vi "Begin.vi"(8 "error in":errorcluster) -> (0 "error out":errorcluster)   [LabVIEW 2014]
doc: "Called before other user functions, this VI is expected to open initial I/O refnums, load in file data, and do all program initialization. Notice that the <B>error out</B> terminal is simply used for data flow. Wiring it to other structures or subVIs ensures that this VI runs first."
uses:
  <vilib>/Rock Robotics/WPI/DriverStation/WPI_DriverStationRobotMode2.ctl
  <vilib>/Rock Robotics/SystemInterfaces/DIO/FPGA_DIOPWMChannel.ctl
  <vilib>/Rock Robotics/WPI/SafetyOutput/WPI_SafetyOutputConfigMenu.ctl
  <vilib>/Rock Robotics/WPI/Joystick/WPI_JoystickDeviceEnum.ctl
  <vilib>/Rock Robotics/SystemInterfaces/DIO/FPGA_DIOChannel.ctl
  <vilib>/Rock Robotics/SystemInterfaces/Typedef/FPGA_TypedefAnalogModuleForGyro.ctl
  <vilib>/Rock Robotics/SystemInterfaces/AI/FPGA_AIGyroChannel.ctl
  <vilib>/Rock Robotics/WPI/Solenoid/WPI_SolenoidChannel.ctl
  <vilib>/Rock Robotics/Network Tables/SD Write String Array.vi
  Robot Global Data.vi
  <vilib>/Rock Robotics/WPI/MotorControl/WPI_MotorControlOpen Talon.vi
  <vilib>/Rock Robotics/WPI/RobotDrive/WPI_RobotDriveOpen4MotorWithTalon.vi
  <vilib>/Rock Robotics/WPI/Counter/WPI_CounterDigitalInputToDigitalSource.vi
  <vilib>/Rock Robotics/WPI/Solenoid/WPI_SolenoidOpenSingle.vi
  <vilib>/Rock Robotics/WPI/Solenoid/WPI_SolenoidOpenDouble.vi
  <vilib>/Rock Robotics/WPI/Compressor/WPI_CompressorGetSetRefNum.vi
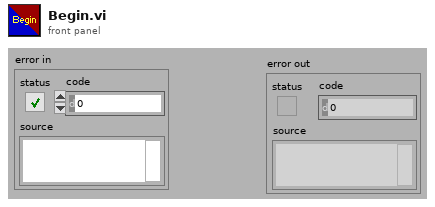
[diagram p1: front panel]
types:
  T1 = typedef "WPI_SolenoidChannel.ctl" = enum8{"Solenoid 0", "Solenoid 1", "Solenoid 2", "Solenoid 3", "Solenoid 4", "Solenoid 5", "Solenoid 6", "Solenoid 7", "Invalid"}
  T2 = typedef "FPGA_DIOChannel.ctl" = enum8{"DIO 0", "DIO 1", "DIO 2", "DIO 3", "DIO 4", "DIO 5", "DIO 6", "DIO 7", "DIO 8", "DIO 9", "DIO MXP 0", "DIO MXP 1", "DIO MXP 2", "DIO MXP 3", "DIO MXP 4", "DIO MXP 5", "DIO MXP 6", "DIO MXP 7", "DIO MXP 8", "DIO MXP 9", "DIO MXP 10", "DIO MXP 11", "DIO MXP 12", "DIO MXP 13", "DIO MXP 14", "DIO MXP 15", "Invalid"}
  T3 = typedef "FPGA_DIOPWMChannel.ctl" = enum8{"PWM 0", "PWM 1", "PWM 2", "PWM 3", "PWM 4", "PWM 5", "PWM 6", "PWM 7", "PWM 8", "PWM 9", "PWM MXP 0", "PWM MXP 1", "PWM MXP 2", "PWM MXP 3", "PWM MXP 4", "PWM MXP 5", "PWM MXP 6", "PWM MXP 7", "PWM MXP 8", "PWM MXP 9", "Invalid"}
  T4 = typedef "FPGA_AIGyroChannel.ctl" = enum8{"AI 0", "AI 1", "Invalid"}
  T5 = typedef "FPGA_TypedefAnalogModuleForGyro.ctl" = enum16{"Controller 1"}
  T6 = typedef "WPI_JoystickDeviceEnum.ctl" = enum16{"USB 0", "USB 1", "USB 2", "USB 3", "USB 4", "USB 5"}
  T7 = typedef "WPI_SafetyOutputConfigMenu.ctl" = enum16{"Enable", "Disable"}
  T8 = typedef "WPI_DriverStationRobotMode2.ctl" = enum16{"Autonomous Disabled", "Autonomous Enabled", "Teleop Disabled", "Teleop Enabled", "Disconnected", "Finish", "Test Disabled", "Test Enabled", "Emergency Stopped"}
  T9 = typedef "WPI_MotorControlDeviceRef.ctl" = cluster{"DeviceStatus":errorcluster, "Type":T10, "PWM":cluster{"Controller":T11, "PWM Channel":T3, "DeadBand":T12}, "CAN":cluster{"Device Number":u8, "Control Mode":T13, "Semaphore":T14, "Max Vout":dbl, "TalonSRX Control Mode":T15}, "Invert":bool, "TransformRef":T16, "InvTransformRef":T16}
  T10 = typedef "WPI_MotorControlType.ctl" = enum16{"PWM", "CAN", "CANTalonSRX"}
  T11 = typedef "FPGA_TypedefDigitalModule.ctl" = enum16{"Controller 1"}
  T12 = typedef "WPI_PWMDeadband.ctl" = cluster{"Name":string, "maxPositivePwm":i32, "minPositivePwm":i32, "centerPwm":i32, "maxNegativePwm":i32, "minNegativePwm":i32, "angularRange":u16}
  T13 = typedef "WPI_CANJaguar_ControlMode.ctl" = enum8{"Percent VBus", "Current", "Speed", "Position", "Voltage"}
  T14 = typedef "Semaphore RefNum" = refnum<k1>
  T15 = typedef "WPI_CANTalonSRX_APIControlMode.ctl" = enum8{"Percent VBus", "Speed", "Position", "Slave", "Unchanged / Invalid"}
  T16 = typedef "WPI_PWMTransform_ConPane.ctl" = refnum<vi>
  T17 = typedef "WPI_CompressorDevRef.ctl" = cluster{"DevStatus":errorcluster, "Pneumatics Control Module":u8}
  T18 = typedef "WPI_DigitalInputDevRef.ctl" = cluster{"DevStatus":errorcluster, "DIO Channel":T2, "Controller":T11}
  T19 = typedef "WPI_JoystickDevRef.ctl" = cluster{"Device":T6}
  T20 = typedef "WPI_SolenoidDevRef.ctl" = cluster{"DevStatus":errorcluster, "Pneumatics Control Module":u8, "Forward Solenoid Channel":T1, "Reverse Solenoid Channel":T1}
  T21 = typedef "WPI_GyroDevRef.ctl" = cluster{"DevStatus":errorcluster, "Analog Module":T22, "Analog Channel":T23, "Offset":dbl, "Gain (VoltsPerDegree/Second)":dbl}
  T22 = typedef "FPGA_TypedefAnalogModule.ctl" = enum16{"Controller 1"}
  T23 = typedef "FPGA_AIChannel.ctl" = enum8{"AI 0", "AI 1", "AI 2", "AI 3", "AI MXP 0", "AI MXP 1", "AI MXP 2", "AI MXP 3", "Invalid"}
  T24 = typedef "FPGA_CounterEncoderSourceConvertionLVSourceType.ctl" = cluster{"DevStatus":errorcluster, "AnalogTriggerMode?":bool, "DigitalMode":cluster{"Controller":T11, "DIO Channel":T25}, "AnalogTriggerMode":cluster{"AnalogTriggerIndex":T26, "OutputType":T27}}
  T25 = typedef "FPGA_DIODigitalSourceChannel.ctl" = enum8{"DIO 0", "DIO 1", "DIO 2", "DIO 3", "DIO 4", "DIO 5", "DIO 6", "DIO 7", "DIO 8", "DIO 9", "DIO MXP 0", "DIO MXP 1", "DIO MXP 2", "DIO MXP 3", "DIO MXP 4", "DIO MXP 5", "DIO MXP 6", "DIO MXP 7", "DIO MXP 8", "DIO MXP 9", "DIO MXP 10", "DIO MXP 11", "DIO MXP 12", "DIO MXP 13", "DIO MXP 14", "DIO MXP 15", "Disabled"}
  T26 = typedef "FPGA_AnalogTriggerIndex.ctl" = enum8{"Trig 0", "Trig 1", "Trig 2", "Trig 3", "Trig 4", "Trig 5", "Trig 6", "Trig 7", "Invalid"}
  T27 = typedef "FPGA_AnalogTriggerOutType.ctl" = enum16{"InWindow", "TriggerState", "Rising", "Falling"}
  T28 = typedef "WPI_RobotDriveDevRef.ctl" = cluster{"DevStatus":errorcluster, "Motors[]":T9[], "Square Inputs":bool, "Max Output":dbl}
  T29 = typedef "WPI_EncoderDevRef.ctl" = cluster{"DevStatus":errorcluster, "EncoderIndex":T30, "CounterIndex":T31, "DistancePerCount":dbl, "Decoding Type":T32}
  T30 = typedef "FPGA_EncoderIdx.ctl" = enum8{"Enc 0", "Enc 1", "Enc 2", "Enc 3", "Enc 4", "Enc 5", "Enc 6", "Enc 7", "Invalid"}
  T31 = typedef "FPGA_CounterCtrSystemIndex.ctl" = enum8{"Ctr 0", "Ctr 1", "Ctr 2", "Ctr 3", "Ctr 4", "Ctr 5", "Ctr 6", "Ctr 7", "Invalid"}
  T32 = typedef "WPI_EncoderType.ctl" = enum16{"1x", "2x", "4x"}
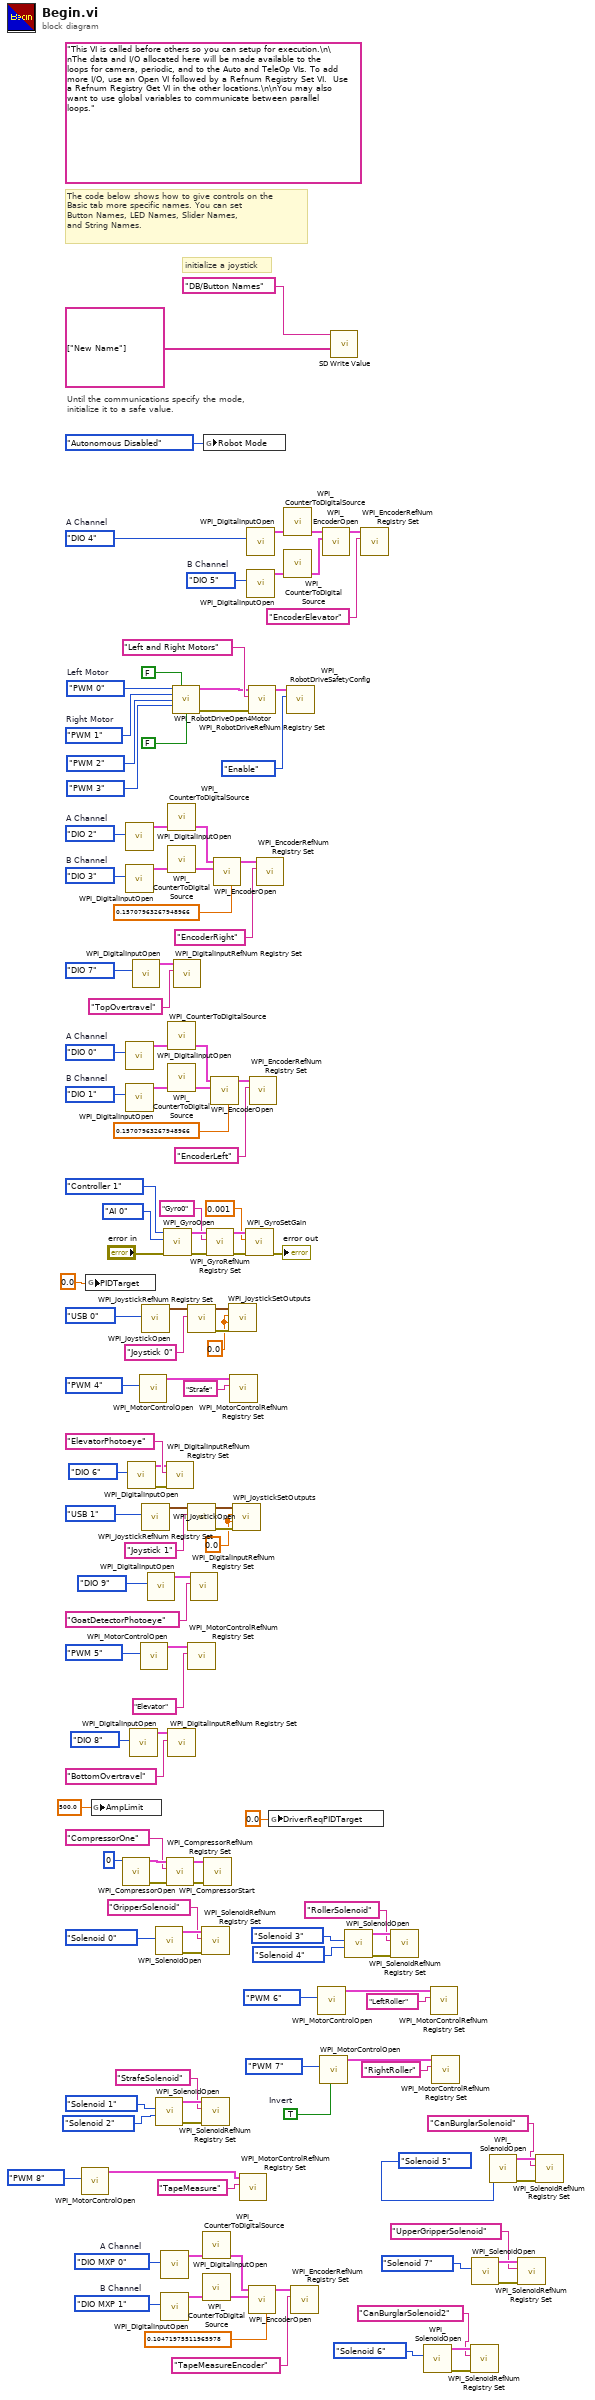
[diagram p0: block diagram]
diagram:
  w10 = 0.0
  w11 = 0.0
  w20 = FPGA_DIOChannel."DIO MXP 1"  # B Channel
  w21 = FPGA_DIOChannel."DIO MXP 0"  # A Channel
  w31 = TRUE  # Invert
  w118 = FPGA_DIOChannel."DIO 5"  # B Channel
  w119 = FPGA_DIOChannel."DIO 4"  # A Channel
  w111 = FPGA_DIOChannel."DIO 3"  # B Channel
  w112 = FPGA_DIOChannel."DIO 2"  # A Channel
  w103 = FPGA_DIOChannel."DIO 1"  # B Channel
  w104 = FPGA_DIOChannel."DIO 0"  # A Channel
  w84 = FPGA_DIOPWMChannel."PWM 1"  # Right Motor
  w83 = FPGA_DIOPWMChannel."PWM 0"  # Left Motor
  (unwired) "This VI is called before others so you can setup for execution.\n\nThe data and I/O allocated here will be made available to the loops for camera, periodic, and to the Auto and TeleOp VIs. To add more I/O, use an Open VI followed by a Refnum Registry Set VI.  Use a Refnum Registry Get VI in the other locations.\n\nYou may also want to use global variables to communicate between parallel loops."
  # "The code below shows how to give controls on the\nBasic tab more specific names. You can set\nButton Names, LED Names, Slider Names,\nand String Names."
  # "initialize a joystick"
  # "Until the communications specify the mode,\ninitialize it to a safe value."
  n1 = call-poly <vilib>:"WPI_MotorControlOpen.vi"("PWM Channel"=FPGA_DIOPWMChannel."PWM 8") -> ("MotorControlDeviceRef"=w28:T9)  [unwired: 9 in, 1 out]
  n2 = global write "Robot Global Data.vi" "PIDTarget"(0.0 ("PIDTarget")) -> ()
  n3 = global write "Robot Global Data.vi" "AmpLimit"(500.0 ("AmpLimit")) -> ()
  n4 = call <vilib>:"WPI_CompressorOpen.vi"("Pneumatics Control Module (0)"=u8 0) -> ("CompressorDevRef"=w62:T17, "error out"=w59:errorcluster)  [unwired: 13 in]
  n5 = call <vilib>:"WPI_DigitalInputOpen.vi"("DIO Channel"=w112) -> ("DigitalInputDevRef"=w115:T18)  [unwired: 2 in, 8 out]
  n6 = call <vilib>:"WPI_DigitalInputOpen.vi"("DIO Channel"=w111) -> ("DigitalInputDevRef"=w114:T18)  [unwired: 2 in, 8 out]
  n7 = call <vilib>:"WPI_DigitalInputOpen.vi"("DIO Channel"=w104) -> ("DigitalInputDevRef"=w107:T18)  [unwired: 2 in, 8 out]
  n8 = call <vilib>:"WPI_DigitalInputOpen.vi"("DIO Channel"=w103) -> ("DigitalInputDevRef"=w106:T18)  [unwired: 2 in, 8 out]
  n9 = call <vilib>:"WPI_DigitalInputOpen.vi"("DIO Channel"=FPGA_DIOChannel."DIO 6") -> ("error out"=w128:errorcluster, "DigitalInputDevRef"=w129:T18)  [unwired: 9 in]
  n10 = call <vilib>:"WPI_DigitalInputOpen.vi"("DIO Channel"=FPGA_DIOChannel."DIO 8") -> ("DigitalInputDevRef"=w67:T18)  [unwired: 9 in, 1 out]
  n11 = call <vilib>:"WPI_DigitalInputOpen.vi"("DIO Channel"=FPGA_DIOChannel."DIO 7") -> ("DigitalInputDevRef"=w69:T18)  [unwired: 9 in, 1 out]
  n12 = call-poly <vilib>:"WPI_MotorControlOpen.vi"("PWM Channel"=FPGA_DIOPWMChannel."PWM 4") -> ("MotorControlDeviceRef"=w93:T9)  [unwired: 9 in, 1 out]
  n13 = call-poly <vilib>:"WPI_MotorControlOpen.vi"("PWM Channel"=FPGA_DIOPWMChannel."PWM 5") -> ("MotorControlDeviceRef"=w98:T9)  [unwired: 9 in, 1 out]
  n14 = call <vilib>:"WPI_JoystickOpen.vi"("JoystickDevice"=WPI_JoystickDeviceEnum."USB 0") -> ("JoystickDevRef"=w88:T19)  [unwired: 10 in]
  n15 = call <vilib>:"WPI_JoystickOpen.vi"("JoystickDevice"=WPI_JoystickDeviceEnum."USB 1") -> ("JoystickDevRef"=w101:T19)  [unwired: 10 in]
  n16 = call <vilib>:"WPI_DigitalInputOpen.vi"("DIO Channel"=FPGA_DIOChannel."DIO 9") -> ("DigitalInputDevRef"=w51:T18)  [unwired: 9 in, 1 out]
  n17 = call-poly <vilib>:"WPI_SolenoidOpen.vi"("Solenoid Channel"=WPI_SolenoidChannel."Solenoid 0") -> ("error out"=w61:errorcluster, "SolenoidDevRef"=w60:T20)  [unwired: 9 in]
  n18 = call-poly <vilib>:"WPI_SolenoidOpen.vi"("Reverse Solenoid Channel"=WPI_SolenoidChannel."Solenoid 2" ("Solenoid Channel"), "Forward Solenoid Channel"=WPI_SolenoidChannel."Solenoid 1" ("Solenoid Channel")) -> ("error out"=w48:errorcluster, "SolenoidDevRef"=w47:T20)  [unwired: 8 in]
  n19 = call <vilib>:"WPI_DigitalInputOpen.vi"("DIO Channel"=w21) -> ("DigitalInputDevRef"=w24:T18)  [unwired: 2 in, 8 out]
  n20 = call <vilib>:"WPI_DigitalInputOpen.vi"("DIO Channel"=w20) -> ("DigitalInputDevRef"=w23:T18)  [unwired: 2 in, 8 out]
  n21 = call <vilib>:"WPI_GyroOpen.vi"("error in (no error)"="error in", "Analog Channel"=FPGA_AIGyroChannel."AI 0", "Controller"=FPGA_TypedefAnalogModuleForGyro."Controller 1") -> ("error out"=w77:errorcluster, "GyroDevRef"=w76:T21)  [unwired: 6 in, 1 out]
  n22 = call <vilib>:"WPI_DigitalInputRefNum Registry Set.vi"("error in (no error)"=w128, "refnum name"="ElevatorPhotoeye", "DigitalInputDevRef"=w129) -> ()  [unwired: 7 in, 2 out]
  n23 = call <vilib>:"WPI_CompressorRefNum Registry Set.vi"("error in (no error)"=w59, "refnum name"="CompressorOne", "CompressorDevRef"=w62) -> ("error out"=w55:errorcluster, "CompressorDevRef"=w56:T17)  [unwired: 7 in]
  n24 = call-poly <vilib>:"WPI_CounterToDigitalSource.vi"("DigitalInputDevRef"=w115) -> ("Digital Source"=w116:T24)  [unwired: 6 out]
  n25 = call-poly <vilib>:"WPI_CounterToDigitalSource.vi"("DigitalInputDevRef"=w114) -> ("Digital Source"=w113:T24)  [unwired: 6 out]
  n26 = call-poly <vilib>:"WPI_CounterToDigitalSource.vi"("DigitalInputDevRef"=w107) -> ("Digital Source"=w108:T24)  [unwired: 6 out]
  n27 = call-poly <vilib>:"WPI_CounterToDigitalSource.vi"("DigitalInputDevRef"=w106) -> ("Digital Source"=w105:T24)  [unwired: 6 out]
  n28 = call <vilib>:"WPI_DigitalInputRefNum Registry Set.vi"("refnum name"="BottomOvertravel", "DigitalInputDevRef"=w67) -> ()  [unwired: 8 in, 2 out]
  n29 = call-poly <vilib>:"WPI_RobotDriveOpen4Motor.vi"("Rear Left Motor"=w83, "Rear Left Motor Inverted"=FALSE, "Rear Right Motor"=w84, "Front Left Motor"=FPGA_DIOPWMChannel."PWM 2", "Front Right Motor"=FPGA_DIOPWMChannel."PWM 3", "Front Right Motor Inverted"=FALSE) -> ("RobotDriveDevRef"=w80:T28, "error out"=w82:errorcluster)  [unwired: 8 in]
  n30 = call <vilib>:"WPI_DigitalInputRefNum Registry Set.vi"("refnum name"="TopOvertravel", "DigitalInputDevRef"=w69) -> ()  [unwired: 8 in, 2 out]
  n31 = call <vilib>:"WPI_JoystickRefNum Registry Set.vi"("refnum name"="Joystick 0", "JoystickDevRef"=w88) -> ("error out"=w15:errorcluster, "JoystickDevRef"=w14:T19)  [unwired: 8 in]
  n32 = call <vilib>:"WPI_JoystickRefNum Registry Set.vi"("refnum name"="Joystick 1", "JoystickDevRef"=w101) -> ("error out"=w12:errorcluster, "JoystickDevRef"=w13:T19)  [unwired: 8 in]
  n33 = call <vilib>:"WPI_MotorControlRefNum Registry Set.vi"("refnum name"="Elevator", "MotorControlDevRef"=w98) -> ()  [unwired: 8 in, 2 out]
  n34 = call <vilib>:"WPI_DigitalInputRefNum Registry Set.vi"("refnum name"="GoatDetectorPhotoeye", "DigitalInputDevRef"=w51) -> ()  [unwired: 8 in, 2 out]
  n35 = call <vilib>:"WPI_SolenoidRefNum Registry Set.vi"("error in (no error)"=w61, "refnum name"="GripperSolenoid", "SolenoidDevRef"=w60) -> ()  [unwired: 7 in, 2 out]
  n36 = call <vilib>:"WPI_SolenoidRefNum Registry Set.vi"("error in (no error)"=w48, "refnum name"="StrafeSolenoid", "SolenoidDevRef"=w47) -> ()  [unwired: 7 in, 2 out]
  n37 = call-poly <vilib>:"WPI_CounterToDigitalSource.vi"("DigitalInputDevRef"=w24) -> ("Digital Source"=w25:T24)  [unwired: 6 out]
  n38 = call-poly <vilib>:"WPI_CounterToDigitalSource.vi"("DigitalInputDevRef"=w23) -> ("Digital Source"=w22:T24)  [unwired: 6 out]
  n39 = global write "Robot Global Data.vi" "Robot Mode"(WPI_DriverStationRobotMode2."Autonomous Disabled" ("Robot Mode")) -> ()
  n40 = call <vilib>:"WPI_CompressorStart.vi"("error in (no error)"=w55, "CompressorDevRef"=w56) -> ()  [unwired: 8 in, 2 out]
  n41 = call <vilib>:"WPI_GyroRefNum Registry Set.vi"("error in (no error)"=w77, "refnum name"="Gyro0", "GyroDevRef"=w76) -> ("error out"=w75:errorcluster, "GyroDevRef"=w74:T21)  [unwired: 7 in]
  n42 = call <vilib>:"WPI_EncoderOpen.vi"("DistancePerCount"=0.15707963267948966, "BSource"=w105, "ASource"=w108) -> ("EncoderDevRef"=w109:T29)  [unwired: 5 in, 3 out]
  n43 = call <vilib>:"WPI_EncoderOpen.vi"("DistancePerCount"=0.15707963267948966, "BSource"=w113, "ASource"=w116) -> ("EncoderDevRef"=w117:T29)  [unwired: 5 in, 3 out]
  n44 = call <vilib>:"WPI_JoystickSetOutputs.vi"("error in (no error)"=w15, "Right Rumble"=w10, "Left Rumble"=w10, "JoystickDevRef"=w14) -> ()  [unwired: 6 in, 2 out]
  n45 = call <vilib>:"WPI_MotorControlRefNum Registry Set.vi"("refnum name"="Strafe", "MotorControlDevRef"=w93) -> ()  [unwired: 8 in, 2 out]
  n46 = call <vilib>:"WPI_JoystickSetOutputs.vi"("error in (no error)"=w12, "Right Rumble"=w11, "Left Rumble"=w11, "JoystickDevRef"=w13) -> ()  [unwired: 6 in, 2 out]
  n47 = call <vilib>:"WPI_MotorControlRefNum Registry Set.vi"("refnum name"="TapeMeasure", "MotorControlDevRef"=w28) -> ()  [unwired: 8 in, 2 out]
  n48 = call <vilib>:"WPI_GyroSetGain.vi"("error in (no error)"=w75, "Gain (VoltsPerDegree/Second)"=0.001, "GyroDevRef"=w74) -> ("error out"=→"error out":errorcluster)  [unwired: 7 in, 1 out]
  n49 = call <vilib>:"WPI_DigitalInputOpen.vi"("DIO Channel"=w119) -> ("DigitalInputDevRef"=w122:T18)  [unwired: 2 in, 8 out]
  n50 = call <vilib>:"WPI_DigitalInputOpen.vi"("DIO Channel"=w118) -> ("DigitalInputDevRef"=w121:T18)  [unwired: 2 in, 8 out]
  n51 = call <vilib>:"WPI_RobotDriveRefNum Registry Set.vi"("error in (no error)"=w82, "refnum name"="Left and Right Motors", "RobotDriveDevRef"=w80) -> ("RobotDriveDevRef"=w85:T28)  [unwired: 8 out]
  n52 = call <vilib>:"WPI_EncoderOpen.vi"("DistancePerCount"=0.10471975511965978, "BSource"=w22, "ASource"=w25) -> ("EncoderDevRef"=w26:T29)  [unwired: 5 in, 3 out]
  n53 = call <vilib>:"WPI_EncoderRefNum Registry Set.vi"("refnum name"="EncoderLeft", "EncoderDevRef"=w109) -> ()  [unwired: 8 in, 2 out]
  n54 = call <vilib>:"WPI_EncoderRefNum Registry Set.vi"("refnum name"="EncoderRight", "EncoderDevRef"=w117) -> ()  [unwired: 8 in, 2 out]
  n55 = global write "Robot Global Data.vi" "DriverReqPIDTarget"(0.0 ("DriverReqPIDTarget")) -> ()
  n56 = call-poly <vilib>:"WPI_CounterToDigitalSource.vi"("DigitalInputDevRef"=w122) -> ("Digital Source"=w123:T24)  [unwired: 6 out]
  n57 = call-poly <vilib>:"WPI_CounterToDigitalSource.vi"("DigitalInputDevRef"=w121) -> ("Digital Source"=w120:T24)  [unwired: 6 out]
  n58 = call <vilib>:"WPI_RobotDriveSafetyConfig.vi"("mode"=WPI_SafetyOutputConfigMenu."Enable", "RobotDriveDevRef"=w85) -> ()  [unwired: 8 in, 2 out]
  n59 = call <vilib>:"WPI_EncoderRefNum Registry Set.vi"("refnum name"="TapeMeasureEncoder", "EncoderDevRef"=w26) -> ()  [unwired: 8 in, 2 out]
  n60 = call-poly <vilib>:"WPI_MotorControlOpen.vi"("PWM Channel"=FPGA_DIOPWMChannel."PWM 6") -> ("MotorControlDeviceRef"=w37:T9)  [unwired: 9 in, 1 out]
  n61 = call-poly <vilib>:"WPI_MotorControlOpen.vi"("Invert"=w31, "PWM Channel"=FPGA_DIOPWMChannel."PWM 7") -> ("MotorControlDeviceRef"=w34:T9)  [unwired: 8 in, 1 out]
  n62 = call <vilib>:"WPI_EncoderOpen.vi"("BSource"=w120, "ASource"=w123) -> ("EncoderDevRef"=w124:T29)  [unwired: 6 in, 3 out]
  n63 = call-poly <vilib>:"SD Write Value.vi"("String Array"=string[] ["New Name"], "Name"="DB/Button Names") -> ()  [unwired: 8 in, 2 out]
  n64 = call-poly <vilib>:"WPI_SolenoidOpen.vi"("Reverse Solenoid Channel"=WPI_SolenoidChannel."Solenoid 4", "Forward Solenoid Channel"=WPI_SolenoidChannel."Solenoid 3" ("Solenoid Channel")) -> ("error out"=w42:errorcluster, "SolenoidDevRef"=w41:T20)  [unwired: 8 in]
  n65 = call <vilib>:"WPI_EncoderRefNum Registry Set.vi"("refnum name"="EncoderElevator", "EncoderDevRef"=w124) -> ()  [unwired: 8 in, 2 out]
  n66 = call <vilib>:"WPI_SolenoidRefNum Registry Set.vi"("error in (no error)"=w42, "refnum name"="RollerSolenoid", "SolenoidDevRef"=w41) -> ()  [unwired: 7 in, 2 out]
  n67 = call-poly <vilib>:"WPI_SolenoidOpen.vi"("Solenoid Channel"=WPI_SolenoidChannel."Solenoid 6") -> ("error out"=w4:errorcluster, "SolenoidDevRef"=w3:T20)  [unwired: 9 in]
  n68 = call <vilib>:"WPI_MotorControlRefNum Registry Set.vi"("refnum name"="LeftRoller", "MotorControlDevRef"=w37) -> ()  [unwired: 8 in, 2 out]
  n69 = call <vilib>:"WPI_MotorControlRefNum Registry Set.vi"("refnum name"="RightRoller", "MotorControlDevRef"=w34) -> ()  [unwired: 8 in, 2 out]
  n70 = call <vilib>:"WPI_SolenoidRefNum Registry Set.vi"("error in (no error)"=w4, "refnum name"="CanBurglarSolenoid2", "SolenoidDevRef"=w3) -> ()  [unwired: 7 in, 2 out]
  n71 = call-poly <vilib>:"WPI_SolenoidOpen.vi"("Solenoid Channel"=WPI_SolenoidChannel."Solenoid 7") -> ("error out"=w9:errorcluster, "SolenoidDevRef"=w8:T20)  [unwired: 9 in]
  n72 = call-poly <vilib>:"WPI_SolenoidOpen.vi"("Solenoid Channel"=WPI_SolenoidChannel."Solenoid 5") -> ("error out"=w18:errorcluster, "SolenoidDevRef"=w17:T20)  [unwired: 9 in]
  n73 = call <vilib>:"WPI_SolenoidRefNum Registry Set.vi"("error in (no error)"=w9, "refnum name"="UpperGripperSolenoid", "SolenoidDevRef"=w8) -> ()  [unwired: 7 in, 2 out]
  n74 = call <vilib>:"WPI_SolenoidRefNum Registry Set.vi"("error in (no error)"=w18, "refnum name"="CanBurglarSolenoid", "SolenoidDevRef"=w17) -> ()  [unwired: 7 in, 2 out]
